vi "NI VeriStand - Get Item Reference by Name.vi"(8 "error in (no error)":errorcluster, 10 "Item Name":string, 11 "Parent Ref in":T1 format="%.0x") -> (0 "error out":errorcluster, 2 "Item Ref":T1 format="%.0x", 3 "Parent Ref out":T1 format="%.0x", 4 "Found":bool)   [LabVIEW 2026, in "Custom Devices Storage.lvlib"]
uses:
  Custom Devices Storage.lvlib
  <vilib>/NI VeriStand/Custom Device API/Custom Device Item Ref.ctl
  C:/Users/Administrator/Desktop/Jatin/All DNC DLLs/NationalInstruments.VeriStand.SystemDefinitionAPI.dll
  Jatin/All DNC DLLs/NationalInstruments.VeriStand.SystemDefinitionAPI.dll
  <vilib>/NI VeriStand/Custom Device API/Custom Device API.lvlib
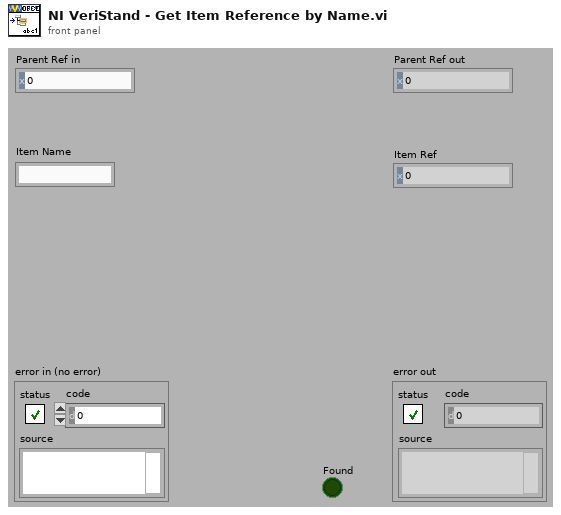
[diagram p1: front panel]
types:
  T1 = typedef "Custom Device API.lvlib/Custom Device Item Ref.ctl" = u64
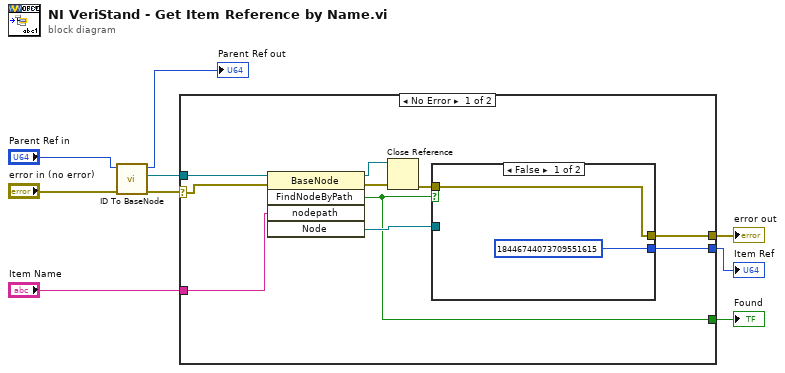
[diagram p0: block diagram]
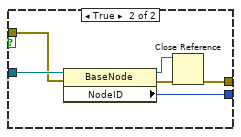
[diagram p2: hidden frame]
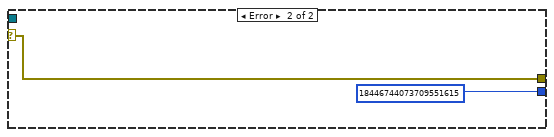
[diagram p3: hidden frame]
diagram:
  n1 = call "ID To BaseNode.vi"("error in (no error)"="error in (no error)", "ID in"="Parent Ref in") -> ("error out"=w9:errorcluster, "NationalInstruments.VeriStand.SystemDefinitionAPI.BaseNode"=w8:refnum<k39>, "ID out"=→"Parent Ref out":u64)  [unwired: 7 in]
  n2 = case shown="No Error" w9 {
    selector: w9 -> [w18 w29]
    tunnel: w8 -> [w19 _]
    tunnel: "Item Name" -> [w17 _]
    tunnel: [w12 T1 18446744073709551615 ("Item Ref")] -> w4
    tunnel: [w11 w29] -> w2
    tunnel: [w10 _] -> w1
    frame No Error {
      n3 = invoke class="BaseNode" method="FindNodeByPath"(reference=w19, error in=w18, "nodepath"=w17) -> (reference out=w15:refnum<k39>, error out=w16:errorcluster, "FindNodeByPath"=w10:bool, "Node"=w14:refnum<k39>)  [unwired: 2 in, 1 out]
      n4 = Close Reference(reference=w15, error in (no error)=w16) -> (error out=w13:errorcluster)
      n5 = case shown="False" w10 {
        tunnel: w14 -> [_ w27]
        tunnel: w13 -> [w20 w26]
        tunnel: [T1 18446744073709551615 ("Item Ref") w23] -> w12
        tunnel: [w20 w22] -> w11
        frame False {
        }
        frame True {
          n6 = property class="BaseNode"(reference=w27, error in=w26) -> (reference out=w24:refnum<k39>, error out=w25:errorcluster, "NodeID"=w23:u64)
          n7 = Close Reference(reference=w24, error in (no error)=w25) -> (error out=w22:errorcluster)
        }
      }
    }
    frame Error {
    }
  }
  "error out" <- w2
  "Found" <- w1
  "Item Ref" <- w4
